vi "write_attributes.vi"(8 "error in (no error)":errorcluster, 10 "attributes":T1, 11 "BaggingRegressor in":refnum<class "BaggingRegressor.lvclass">) -> (0 "error out":errorcluster, 3 "BaggingRegressor out":refnum<class "BaggingRegressor.lvclass">)   [LabVIEW 2020, in "BaggingRegressor.lvclass"]
uses:
  BaggingRegressor.lvclass
  Controls/bagging_regressor_attributes.ctl
  BaggingRegressor.lvclass/BaggingRegressor.ctl
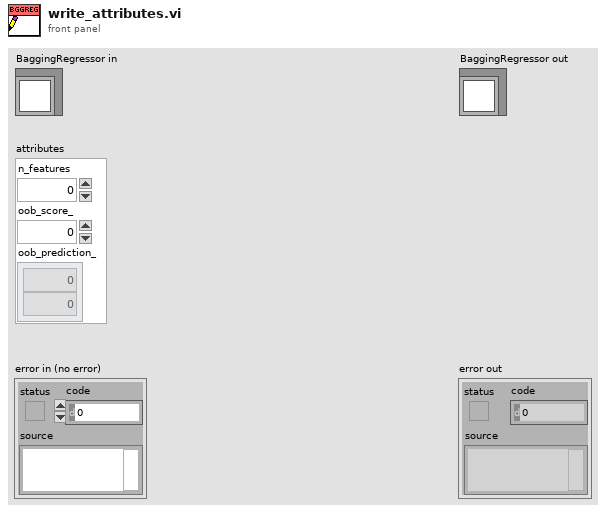
[diagram p1: front panel]
types:
  T1 = typedef "bagging_regressor_attributes.ctl" = cluster{"n_features":dbl, "oob_score_":dbl, "oob_prediction_":dbl[]}
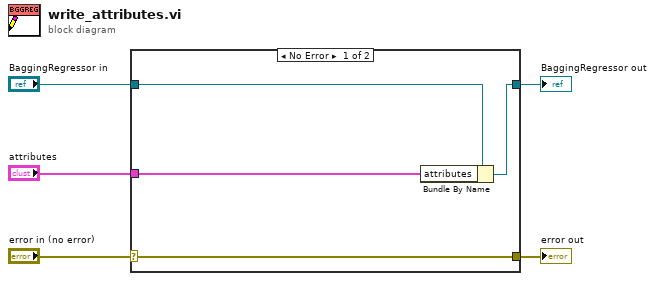
[diagram p0: block diagram]
diagram:
  n1 = case shown="No Error" "error in (no error)" {
    selector: "error in (no error)" -> [w9 w10]
    tunnel: [w9 w10] -> w4
    tunnel: [w7 w11] -> w2
    tunnel: "BaggingRegressor in" -> [w8 w11]
    tunnel: "attributes" -> [w6 _]
    frame No Error {
      n2 = Bundle By Name(cluster=w8, "attributes"=w6) -> (w7:refnum<class "BaggingRegressor.lvclass">)
    }
    frame Error {
    }
  }
  "error out" <- w4
  "BaggingRegressor out" <- w2
